vi "WPI_ERRAcquireInvalidPWMChannelIdx.vi"(8 "error in (no error)":errorcluster, 9 "Additional Depth":i32) -> (0 "error in (no error) 2":errorcluster)   [LabVIEW 2017]
doc: "This software is licensed. Open the labview\\readme\\WPI Robotics Library Open Source License.txt file for more information."
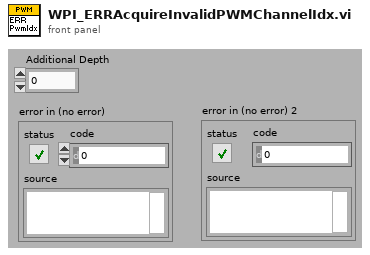
[diagram p1: front panel]
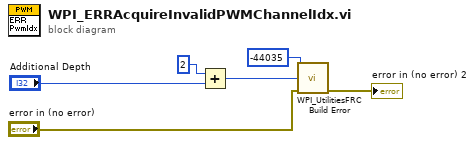
[diagram p0: block diagram]
diagram:
  n1 = Add(x=2 ("chain levels to remove (1)"), y="Additional Depth") -> (x+y=w2:i32)
  n2 = call <vilib>:"WPI_UtilitiesFRC Build Error.vi"("error code"=-44035 ("code"), "chain levels to remove (1)"=w2, "error in (no error)"="error in (no error)") -> ("error out"=→"error in (no error) 2":errorcluster)  [unwired: 2 in, 10 out]
